vi "Read.vi"(8 "error in (no error)":errorcluster, 11 "navX - SPI in":refnum<class "navX - SPI.lvclass">) -> (0 "error out":errorcluster, 3 "navX - SPI out":refnum<class "navX - SPI.lvclass">)   [LabVIEW 2015, in "navX Library v3.lvlib" / "navX - SPI.lvclass"]
uses:
  navX - SPI.lvclass
  navX - Base/navX - Base.lvclass
  navX Registry Cache/navX Registry Cache.lvclass
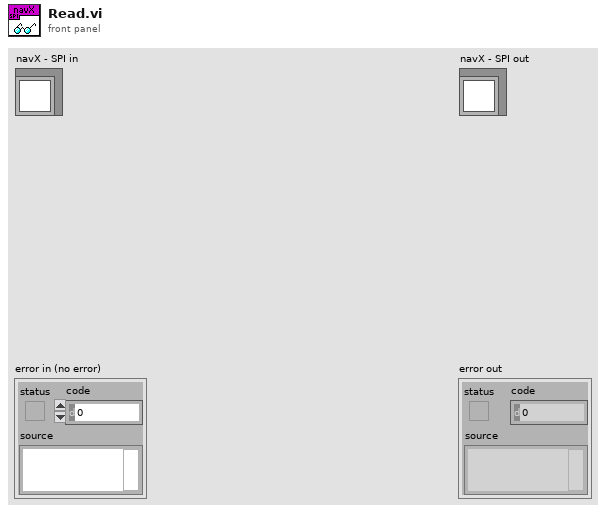
[diagram p1: front panel]
types:
  T1 = typedef "WPI_SPIDevRef.ctl" = cluster{"DevStatus":errorcluster, "Handle":i32, "SPI Bus":T2}
  T2 = typedef "spi_bus.ctl" = enum16{"SPI On-Board, CS0", "SPI On-Board, CS1", "SPI On-Board, CS2", "SPI On-Board, CS3", "SPI MXP", "Invalid"}
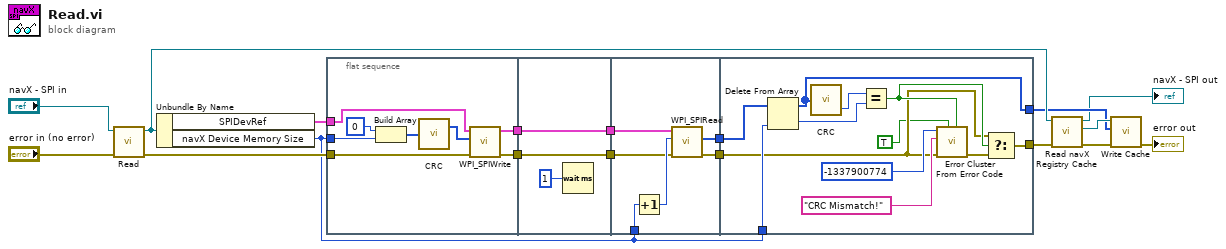
[diagram p0: block diagram]
diagram:
  n1 = call-parent "Read.vi"("error in (no error)"="error in (no error)", "navX - Base in"="navX - SPI in") -> ("error out"=w15:errorcluster, "navX - Base out"=w7:refnum<class "navX - SPI.lvclass">)  [unwired: 8 in]
  n2 = Unbundle By Name(w7) -> ("SPIDevRef"=w16:T1, "navX Device Memory Size"=w8:i32)
  n3 = flat-sequence {
    tunnel: w8 -> [w25]
    tunnel: w16 -> [w22]
    tunnel: w15 -> [w21]
    tunnel: [w20] -> w13
    tunnel: [w19] -> w11
    tunnel: [w28] -> w14
    tunnel: w13 -> [w28]
    tunnel: [w27] -> w12
    tunnel: w11 -> [w27]
    tunnel: w8 -> [w35]
    tunnel: w14 -> [w33]
    tunnel: w12 -> [w32]
    tunnel: [w31] -> w10
    tunnel: [w30] -> w9
    tunnel: w10 -> [w47]
    tunnel: w9 -> [w39]
    tunnel: w8 -> [w46]
    tunnel: [w43] -> w5
    tunnel: [w37] -> w2
    frame #0 {
      n4 = Build Array(u8 0 ("hex"), w25) -> (w24:i32[])
      n5 = call "CRC.vi"("Message"=w24) -> ("Message with CRC"=w23:u8[])  [unwired: 1 out]
      n6 = call <vilib>:"WPI_SPIWrite.vi"("error in (no error)"=w21, "Data To Send"=w23, "SPIDevRef"=w22) -> ("error out"=w19:errorcluster, "SPIDevRef"=w20:T1)  [unwired: 6 in, 1 out]
    }
    frame #1 {
      n7 = Wait (ms)(milliseconds to wait=u32 1) -> ()  [unwired: 1 out]
    }
    frame #2 {
      n8 = Increment(x=w35) -> (x+1=w34:i32)
      n9 = call <vilib>:"WPI_SPIRead.vi"("error in (no error)"=w32, "Num to Read"=w34, "SPIDevRef"=w33) -> ("error out"=w30:errorcluster, "Received Data"=w31:u8[])  [unwired: 6 in, 1 out]
    }
    frame #3 {
      n10 = Delete From Array(array=w47, index=w46) -> (deleted portion=w44:u8, array with subset deleted=w43:u8[])  [unwired: 1 in]
      n11 = call "CRC.vi"("Message"=w43) -> ("CRC"=w45:u8)  [unwired: 1 out]
      n12 = Equal?(x=w45, y=w44) -> (x = y?=w40:bool)
      n13 = call <vilib>:"Error Cluster From Error Code.vi"("is warning? (False)"=w40, "show call chain? (False)"=TRUE, "error in (no error)"=w39, "error message (\"\")"="CRC Mismatch!" ("error message (\"\")"), "error code (0)"=-1337900774) -> ("error out"=w38:errorcluster)  [unwired: 4 in]
      n14 = Select(t=w39, s=w40, f=w38) -> (s? t:f=w37:errorcluster)
    }
  }
  n15 = call "Read navX Registry Cache.vi"("error in (no error)"=w2, "navX - Base in"=w7) -> ("error out"=w1:errorcluster, "navX Library v3.lvlib:navX Registry Cache.lvclass"=w6:refnum<class "navX Registry Cache.lvclass">, "navX - Base out"=→"navX - SPI out":refnum<class "navX - SPI.lvclass">)  [unwired: 7 in]
  n16 = call "Write Cache.vi"("error in (no error)"=w1, "Registry Cache in"=w5, "navX Registry Cache in"=w6) -> ("error out"=→"error out":errorcluster)  [unwired: 7 in, 1 out]
